vi "String to Char Array.vi"(11 "string":string) -> (3 "array of chars":string[](array[string]))   [LabVIEW 2026]
doc: "Convert a string to an arrays of chars."
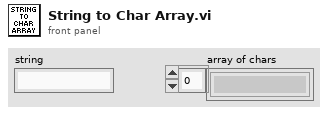
[diagram p1: front panel]
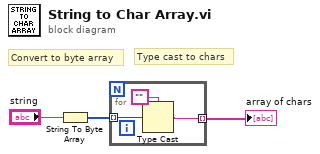
[diagram p0: block diagram]
diagram:
  # "Type cast to chars"
  # "Convert to byte array"
  n1 = String To Byte Array(string="string") -> (unsigned byte array=w3:u8[])
  n2 = for {
    tunnel: w3 -> [w6] mode=indexing
    tunnel: [w4] -> w1 mode=indexing
    n3 = Type Cast(type="", x=w6) -> (*(type *) &x=w4:string)
  }
  "array of chars" <- w1
